vi "image to intermec 'six bits per byte' format.vi"(11 "image data":T1) -> (3 "six bits per byte":string)   [LabVIEW 2018]
uses:
  <vilib>/picture/picture.llb/imagedata.ctl
panel:
  out "output array":bool[][](array[boolean])
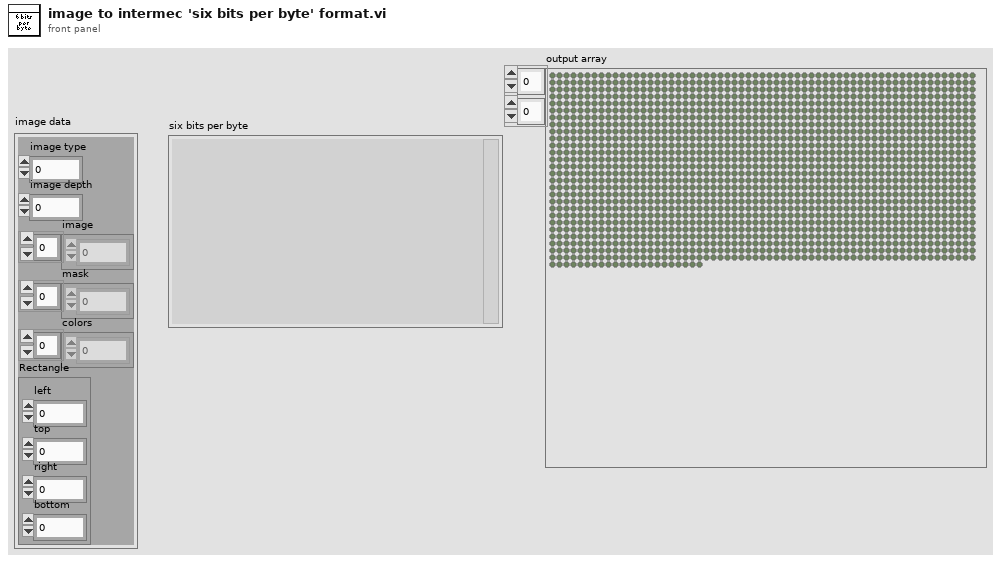
[diagram p1: front panel]
types:
  T1 = typedef "imagedata.ctl" = cluster{"image type":i32, "image depth":i32, "image":u8[], "mask":u8[], "colors":u32[], "Rectangle":cluster{"left":i16, "top":i16, "right":i16, "bottom":i16}}
  T2 = cluster{"left":i16, "top":i16, "right":i16, "bottom":i16}
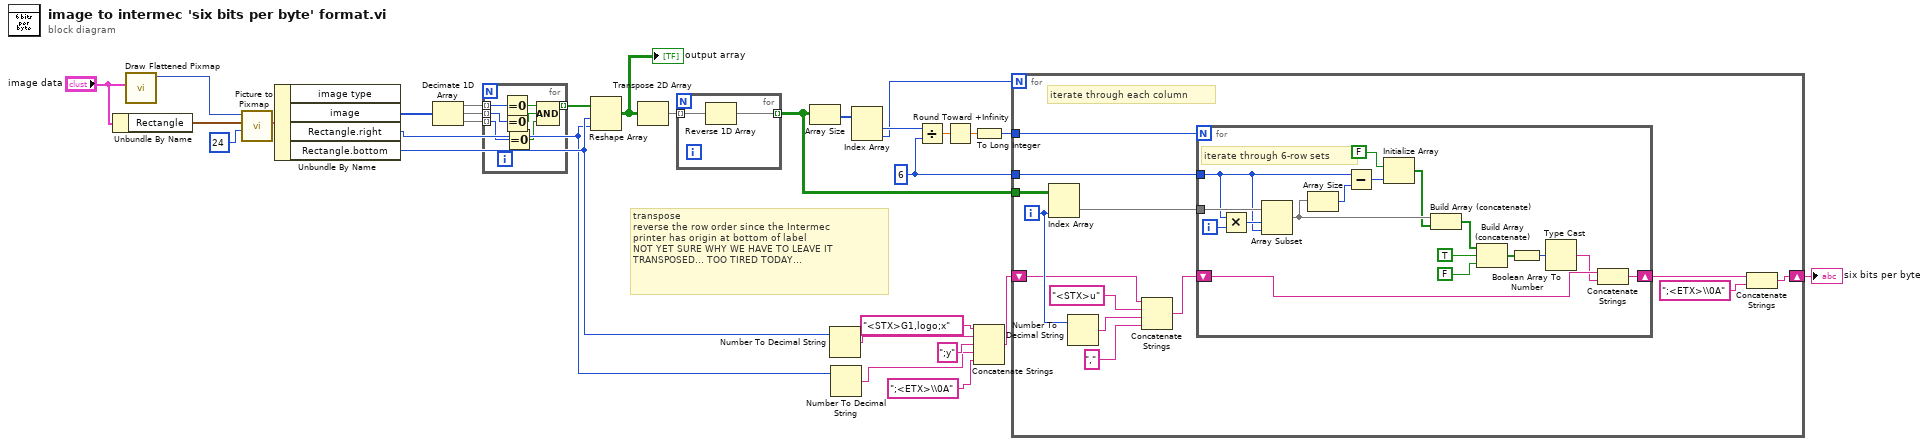
[diagram p0: block diagram]
diagram:
  w22 = 6 ("y")
  # "transpose\nreverse the row order since the Intermec\nprinter has origin at bottom of label\nNOT YET SURE WHY WE HAVE TO LEAVE IT\nTRANSPOSED... TOO TIRED TODAY..."
  n1 = Unbundle By Name("image data") -> ("Rectangle"=w3:T2)
  n2 = call <vilib>:"Draw Flattened Pixmap.vi"("image data"="image data") -> ("new picture"=w7:picture)  [unwired: 8 in]
  n3 = call <vilib>:"Picture to Pixmap.vi"("depth"=24, "rect"=w3, "picture"=w7) -> ("image data"=w5:T1)  [unwired: 7 in, 1 out]
  n4 = Unbundle By Name(w5) -> ("image"=w28:u8[], "Rectangle.right"=w8:i16, "Rectangle.bottom"=w9:i16)  [unwired: 1 out]
  n5 = Decimate 1D Array(w28) -> (w27:u8[], w2:u8[], w1:u8[])
  n6 = for {
    tunnel: [w34] -> w29 mode=indexing
    tunnel: w27 -> [w36] mode=indexing
    tunnel: w2 -> [w33] mode=indexing
    tunnel: w1 -> [w31] mode=indexing
    n7 = Equal To 0?(x=w36) -> (x = 0?=w35:bool)
    n8 = Equal To 0?(x=w33) -> (x = 0?=w32:bool)
    n9 = Equal To 0?(x=w31) -> (x = 0?=w30:bool)
    n10 = Compound Arithmetic op=AND(w35, w32, w30) -> (w34:bool)
  }
  n11 = Reshape Array(w29, w9, w8) -> (w18:bool[][])
  "output array" <- w18
  n12 = Transpose 2D Array(2D array=w18) -> (transposed array=w17:bool[][])
  n13 = for {
    tunnel: w17 -> [w38] mode=indexing
    tunnel: [w37] -> w16 mode=indexing
    n14 = Reverse 1D Array(array=w38) -> (reversed array=w37:bool[])
  }
  n15 = Array Size(array=w16) -> (size(s)=w26:i32[])
  n16 = Number To Decimal String(number=w9) -> (decimal integer string=w11:string)  [unwired: 1 in]
  n17 = Number To Decimal String(number=w8) -> (decimal integer string=w10:string)  [unwired: 1 in]
  n18 = Index Array(array=w26) -> (element #1=w25:i32, element #2=w21:i32)  [unwired: 2 in]
  n19 = Divide(x=w25, y=w22) -> (x/y=w24:dbl)
  n20 = Round Toward +Infinity(x=w24) -> (ceil(x): smallest int >= x=w23:dbl)
  n21 = To Long Integer(number=w23) -> (32bit integer=w20:i32)
  n22 = Concatenate Strings("<STX>G1,logo;x" ("string"), w11, ";y" ("string"), w10, ";<ETX>\\0A" ("string")) -> (w14:string)
  n23 = for {
    N: w21 -> [_]
    tunnel: w16 -> [w50]
    tunnel: w22 -> [w51]
    tunnel: w20 -> [w48]
    shift-right: [w41] -> w19
    shift-left: w14 -> [w40]
    i -> [w47]
    # "iterate through each column"
    n24 = Index Array(array=w50, index (col)=w47) -> (element=w49:bool[])  [unwired: 1 in]
    n25 = Number To Decimal String(number=w47) -> (decimal integer string=w45:string)  [unwired: 1 in]
    n26 = Concatenate Strings(w40, "<STX>u", w45, "," ("string")) -> (w39:string)
    n27 = for {
      N: w48 -> [_]
      tunnel: w49 -> [w68]
      tunnel: w51 -> [w62]
      shift-right: [w59] -> w43
      shift-left: w39 -> [w58]
      i -> [w63]
      # "iterate through 6-row sets"
      n28 = Multiply(x=w62, y=w63) -> (x*y=w64:i32)
      n29 = Array Subset(array=w68, index=w64, length=w62) -> (w67:bool[])
      n30 = Array Size(array=w67) -> (size(s)=w66:i32)
      n31 = Subtract(x=w62, y=w66) -> (x-y=w61:i32)
      n32 = Initialize Array(FALSE, w61) -> (w60:bool[])
      n33 = Build Array (concatenate)(w67, w60) -> (w65:bool[])
      n34 = Build Array (concatenate)(w65, TRUE, FALSE) -> (w52:bool[])
      n35 = Boolean Array To Number(Boolean array=w52) -> (number=w53:u8)
      n36 = Type Cast(x=w53) -> (*(type *) &x=w54:string)  [unwired: 1 in]
      n37 = Concatenate Strings(w58, w54) -> (w59:string)
    }
    n38 = Concatenate Strings(w43, ";<ETX>\\0A") -> (w41:string)
  }
  "six bits per byte" <- w19
